vi "MARS_Plot_Scan_data_wrapper.vi"(4 "1st Int.":i32, 6 "2nd Int":i32, 8 "reference":refnum<vi>, 9 "FoM graph in":dbl[][](array[numeric]), 10 "Total Integral":i32[](array[numeric]), 11 "Tail Integral":i32[](array[numeric])) -> (0 "Histogram":i32[][](graph), 1 "FoM graph out":dbl[][](array[numeric]), 3 "Scan Ratio Graph":i32[][](graph) caption="Intensity Graph")   [LabVIEW 2015]
panel:
  out "FoM":dbl
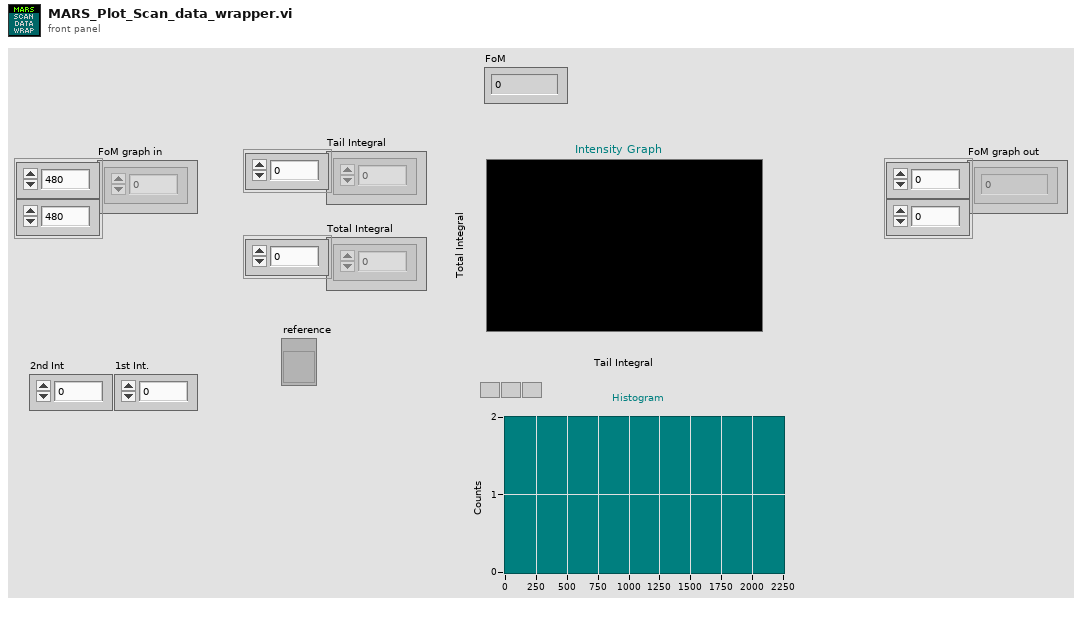
[diagram p1: front panel]
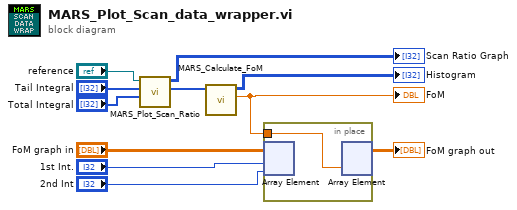
[diagram p0: block diagram]
diagram:
  n1 = call "MARS_Plot_Scan_Ratio.vi"("Total Integral"="Total Integral", "Tail Integral in"="Tail Integral", "IntensityGraph in"="reference") -> ("Histogram"=w7:i32[], "Ratio Graph"=→"Scan Ratio Graph":i32[][])  [unwired: 7 in]
  n2 = call "MARS_Calculate_FoM.vi"("Histogram"=w7) -> ("FoM"=w1:dbl, "Fit Histogram"=→"Histogram":i32[][])  [unwired: 7 in, 2 out]
  "FoM" <- w1
  n3 = in-place {
    in-place-border: w1 -> [w12]
    n4 = in-place-array #1("FoM graph in", "1st Int.", "2nd Int") -> ()  [unwired: 1 out]
    n5 = in-place-array #1(w12) -> (→"FoM graph out":dbl[][])  [unwired: 2 out]
  }
